vi "Create 2D voltage map.vi"(8 "error in (no error)":errorcluster, 10 "1x160  Voltage Map":dbl[](array[numeric]), 11 "BMC in":refnum<class "BMC.lvclass">) -> (0 "error out":errorcluster, 2 "2D Voltage Map":dbl[][](array[numeric]), 3 "BMC out":refnum<class "BMC.lvclass">)   [LabVIEW 2012, in "BMC.lvclass"]
uses:
  BMC.lvclass
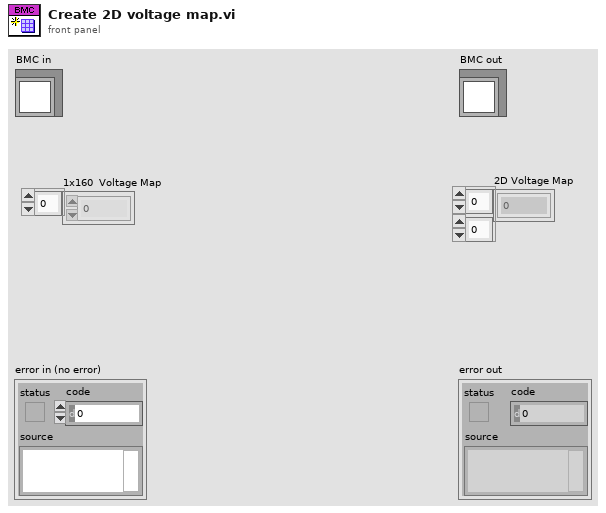
[diagram p1: front panel]
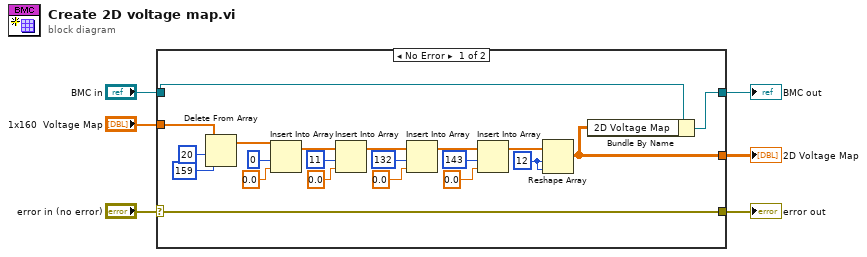
[diagram p0: block diagram]
diagram:
  n1 = case shown="No Error" "error in (no error)" {
    selector: "error in (no error)" -> [w27 w29]
    tunnel: [w27 w29] -> w5
    tunnel: [w9 w28] -> w3
    tunnel: "BMC in" -> [w10 w28]
    tunnel: [w8 _] -> w2
    tunnel: "1x160  Voltage Map" -> [w7 _]
    frame No Error {
      w15 = 12 ("dimension size")
      n2 = Delete From Array(array=w7, length=20, index=159) -> (array with subset deleted=w11:dbl[])  [unwired: 1 out]
      n3 = Insert Into Array(array=w11, index=0, new element=0.0 ("new element/subarray")) -> (w22:dbl[])
      n4 = Insert Into Array(array=w22, index=11, new element=0.0 ("new element/subarray")) -> (w19:dbl[])
      n5 = Insert Into Array(array=w19, index=132, new element=0.0 ("new element/subarray")) -> (w16:dbl[])
      n6 = Insert Into Array(array=w16, index=143, new element=0.0 ("new element/subarray")) -> (w14:dbl[])
      n7 = Reshape Array(w14, w15, w15) -> (w8:dbl[][])
      n8 = Bundle By Name(cluster=w10, "2D Voltage Map"=w8) -> (w9:refnum<class "BMC.lvclass">)
    }
    frame Error {
    }
  }
  "error out" <- w5
  "BMC out" <- w3
  "2D Voltage Map" <- w2
